vi "count rate.vi"() -> ()   [LabVIEW 2014]
doc: "This program takes in data from a Geiger counter, in order to create both a plot of the counts/interval at various times as well as a histogram. The user can select the total time and the interval over which counts should be recorded. The user can also select to omit some points since these are often junk. After counting for the selected time interval the program writes the counts vs time to a file. To create the histogram and best fit the program outputs the counts in an array to two sub vi's.\n\nBryan Ghahremani - SID: 1135515\nKenneth Heide - SID: 1269429"
uses:
  <vilib>/Platform/TimedLoop/XDataNode/timing_clust.ctl
  <vilib>/Platform/TimedLoop/XDataNode/nitl_modes.ctl
  <vilib>/Platform/TimedLoop/XDataNode/wakeup.ctl
  <vilib>/Utility/file.llb/Write To Spreadsheet File (DBL).vi
  <vilib>/platform/TimedLoop/XDataNode/XDataNode.xnode
  <vilib>/Platform/TimedLoop/XDataNode/XDNodeRunTimeDep.lvlib
panel:
  out "Decay Time":dbl=111.38825184198605
  in  "Path to Save":path
  in  "Interval (s)":dbl=1.0
  in  "?":dbl=10.0
  out "Counts vs Time":dynamicdata(graph)=[{"t0"=timestamp(0 s since 1904-01-01), "dt"=1.0, "Y"=[86.0, 89.0, 74.0, 84.0, 95.0, 101.0, 93.0, 90.0, 86.0, 91.0, 94.0, 92.0, 109.0, 103.0, 82.0, 104.0, 102.0, 122.0, 109.0, 94.0, 88.0, 105.0, 89.0, 88.0, 89.0, 85.0, 80.0, 85.0, 86.0, 89.0, 78.0, 102.0, 78.0, 80.0, 85.0, 104.0, 99.0, 81.0, 100.0, 75.0, 74.0, 80.0, 77.0, 77.0, 90.0, 73.0, 92.0, 75.0, 80.0, 80.0, 66.0, 85.0, 100.0, 99.0, 72.0, 59.0, 82.0, 106.0, 72.0, 94.0, 83.0, 70.0, 71.0, 62.0, 74.0, 83.0, 70.0, 77.0, 68.0, 78.0, 66.0, 79.0, 73.0, 79.0, 70.0, 70.0, 68.0, 58.0, 74.0, 64.0, 65.0, 67.0, 66.0, 71.0, 78.0, 55.0, 63.0, 73.0, 62.0, 58.0, 57.0, 60.0, 45.0, 63.0, 61.0, 62.0, 64.0, 56.0, 53.0, 63.0, 67.0, 63.0, 60.0, 63.0, 60.0, 51.0, 52.0, 68.0, 59.0, 50.0, 57.0, 55.0, 54.0, 45.0, 60.0, 55.0, 44.0, 66.0, 55.0, 60.0, 57.0, 53.0, 47.0, 51.0, 56.0, 49.0, 51.0, 61.0, 46.0, 61.0, 50.0, 57.0, 61.0, 47.0, 54.0, 44.0, 52.0, 57.0, 63.0, 56.0, 54.0, 56.0, 44.0, 52.0, 50.0, 48.0, 54.0, 54.0, 40.0, 47.0, 39.0, 38.0, 45.0, 48.0, 52.0, 56.0, 44.0, 47.0, 40.0, 39.0, 49.0, 43.0, 48.0, 52.0, 42.0, 48.0, 57.0, 51.0, 53.0, 34.0, 54.0, 41.0, 39.0, 42.0, 36.0, 53.0, 57.0, 43.0, 54.0, 51.0, 50.0, 56.0, 42.0, 52.0, 45.0, 34.0, 42.0, 52.0, 37.0, 59.0, 53.0, 39.0, 48.0, 46.0, 41.0, 47.0, 45.0, 42.0, 54.0, 44.0, 37.0, 38.0, 52.0, 54.0, 47.0, 44.0, 34.0, 43.0, 43.0, 45.0, 45.0, 40.0, 52.0, 48.0, 39.0, 52.0, 46.0, 49.0, 37.0, 52.0, 44.0, 42.0, 38.0, 43.0, 41.0, 40.0, 57.0, 46.0, 49.0, 39.0, 43.0, 44.0, 36.0, 41.0, 34.0, 36.0, 42.0, 45.0, 37.0, 38.0, 40.0, 52.0, 52.0, 44.0, 44.0, 47.0, 41.0, 44.0, 37.0, 35.0, 56.0, 33.0, 30.0, 41.0, 44.0, 45.0, 39.0, 47.0, 47.0, 44.0, 39.0, 41.0, 35.0, 35.0, 49.0, 59.0, 35.0, 35.0, 51.0, 36.0, 36.0, 36.0, 45.0, 36.0, 39.0, 37.0, 27.0, 35.0, 44.0, 40.0, 44.0, 41.0, 55.0, 38.0, 43.0, 37.0, 43.0, 31.0, 36.0, 28.0, 36.0]}, {"t0"=timestamp(0 s since 1904-01-01), "dt"=1.0, "Y"=array[291 elements], "attributes"=variant("NI_ChannelName"=variant(string "Best fit"))}]
  out "Histogram":dynamicdata(graph)=[{"t0"=timestamp(1 s since 1904-01-01), "dt"=2.0, "Y"=[8.352812174756966e-17, 2.888576339244969e-14, 3.1264302386873654e-12, 1.621526279731439e-10, 4.916216242584155e-09, 9.765499519537962e-08, 1.3685183070826735e-06, 1.4251050451169605e-05, 0.00011459899106855562, 0.0007330223641615576, 0.003818327119683722, 0.016510466629310206, 0.06021002372393977, 0.18767699037711996, 0.505765419365066, 1.1900692662585146, 2.4661763847755136, 4.5352483246952175, 7.451222273498955, 11.003116698148636, 14.682944866992178, 17.79266203324392, 19.666401250935436, 19.907721013027125, 18.524195754366946, 15.898522997565765, 12.625173356480483, 9.303420099997624, 6.378862242077928, 4.079700267706533, 2.4395718972978337, 1.3669389229457132, 0.7191585788466767, 0.3559392398594594, 0.16603084186175723, 0.07311461006202052, 0.030445380630477442, 0.012006094741323943, 0.004490259874679223, 0.0015948669016157635, 0.000538672357019741, 0.00017322419030295564, 5.309903520463841e-05, 1.5532655134751475e-05, 4.340604682793738e-06, 1.1599625212246946e-06, 2.9672298558293295e-07, 7.272405727293939e-08, 1.7092824738259553e-08, 3.855951772431547e-09], "attributes"=variant("NI_ChannelName"=variant(string " (Best fit)"), "NI_ExpIsRelativeTime"=variant(bool TRUE), "NI_ExpStartTimeStamp"=variant(timestamp timestamp(3500690969.465605 s since 1904-01-01)), "NI_ExpTimeStamp"=variant(timestamp timestamp(3500690969.465605 s since 1904-01-01)), "NI_ExpXDimension"=variant(string "BIN"), "NI_OriginalChannelName"=variant(string ""))}, {"t0"=timestamp(1 s since 1904-01-01), "dt"=2.0, "Y"=[0.0, 0.0, 0.0, 0.0, 0.0, 0.0, 0.0, 0.0, 0.0, 0.0, 0.0, 0.0, 0.0, 1.0, 2.0, 1.0, 5.0, 6.0, 21.0, 9.0, 21.0, 8.0, 29.0, 9.0, 15.0, 6.0, 27.0, 5.0, 17.0, 4.0, 12.0, 6.0, 7.0, 2.0, 7.0, 2.0, 9.0, 2.0, 7.0, 2.0, 8.0, 2.0, 8.0, 0.0, 8.0, 1.0, 6.0, 1.0, 0.0, 2.0], "attributes"=variant("NI_ChannelName"=variant(string " (Histogram)"), "NI_ExpIsRelativeTime"=variant(bool TRUE), "NI_ExpStartTimeStamp"=variant(timestamp timestamp(3500690969.465605 s since 1904-01-01)), "NI_ExpTimeStamp"=variant(timestamp timestamp(3500690969.465605 s since 1904-01-01)), "NI_ExpXDimension"=variant(string "BIN"), "NI_OriginalChannelName"=variant(string ""))}]
  in  "Time(s)":dbl=300.0
  out "counts per x second(s)":dbl(knob)=36.0 scale=0.0..100.0
  in  "stop":bool
  # "Omitted initial points"
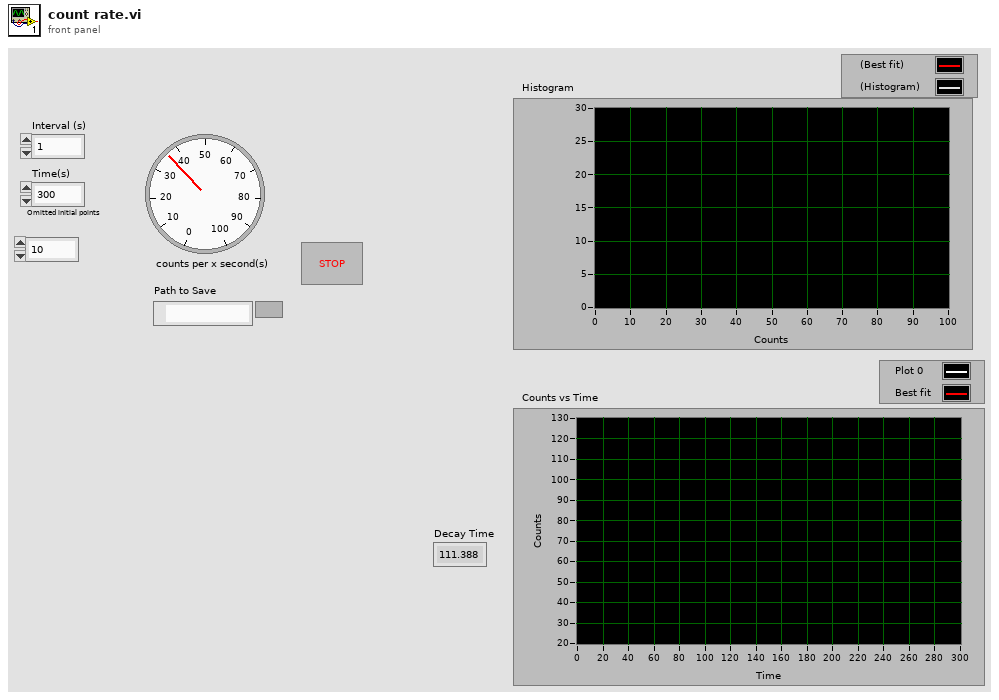
[diagram p1: front panel]
types:
  T1 = typedef "XDNodeRunTimeDep.lvlib/timing_clust.ctl" = cluster{"Expected End [f-1]":u64, "Actual End [f-1]":u64, "Finished Late? [f-1]":bool, "Expected End [i-1]":u64, "Actual End [i-1]":u64, "Finished Late? [i-1]":bool, "Expected Start [i]":u64, "Actual Start [i]":u64, "Expected Start [f]":u64, "Actual Start [f]":u64, "Source Name":string, "Structure Name":string, "Period":i64, "Deadline":i64, "Offset":i64, "Start":i64, "Priority":i32, "Timeout":i32, "Mode":T2, "Wakeup Reason":T3, "Error":errorcluster, "Source Type":string, "Secondary Source Type":string, "Global End Time":u64, "Global Start Time":u64, "Frame Duration":u64, "Iteration Duration":u64, "Assigned CPU":i32, "I/O Scan Engine Mode":u32}
  T2 = typedef "XDNodeRunTimeDep.lvlib/nitl_modes.ctl" = enum32{"No Change", "Process missed periods, maintain original phase", "Discard missed periods, maintain original phase", "Process missed periods, ignore original phase", "Discard missed periods, ignore original phase"}
  T3 = typedef "XDNodeRunTimeDep.lvlib/wakeup.ctl" = enum32{"Normal", "Aborted", "Asynchronous wakeup", "Timing source error", "Timed loop error", "Timeout"}
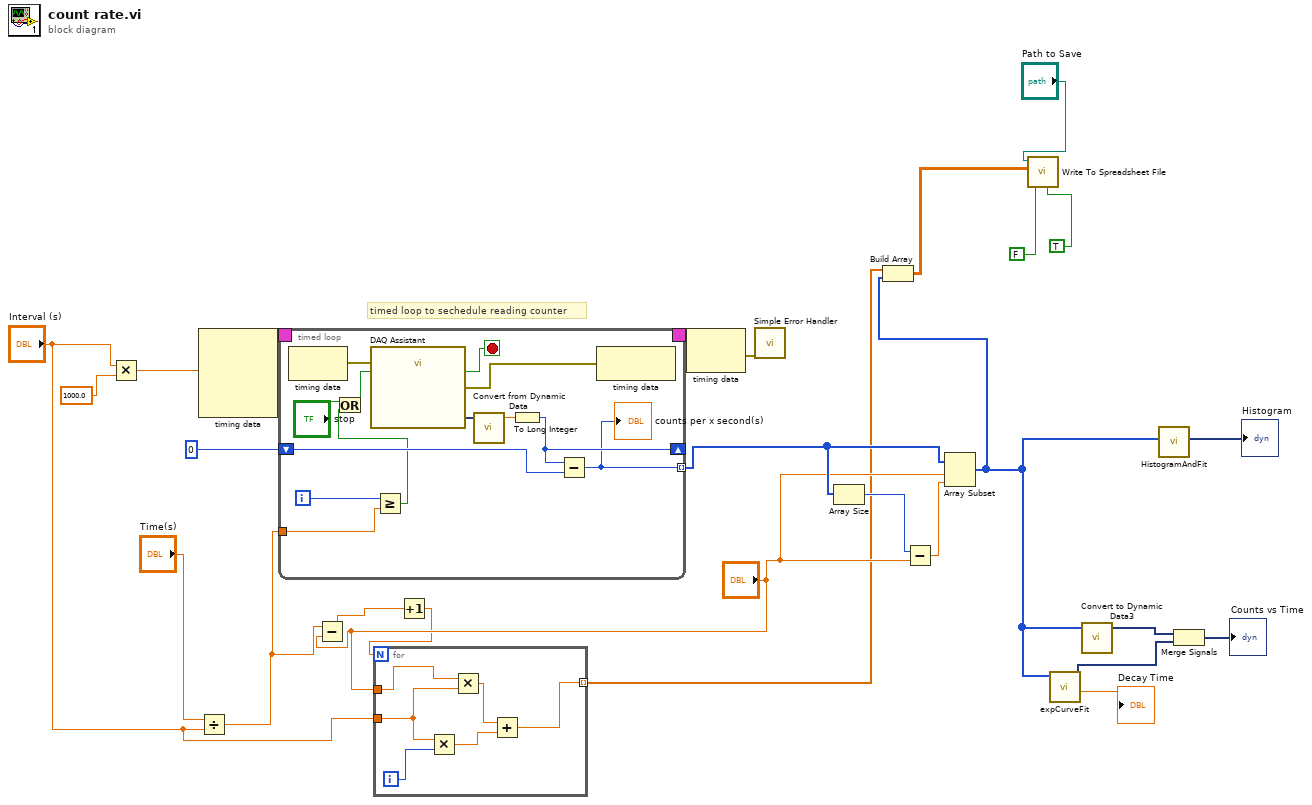
[diagram p0: block diagram]
diagram:
  # "timed loop to sechedule reading counter"
  n1 = Multiply(x="Interval (s)", y=1000.0) -> (x*y=w16:dbl)
  n2 = node-c288(w16) -> (w26:T1)  [unwired: 3 in]
  n3 = Divide(x="Time(s)", y="Interval (s)") -> (x/y=w8:dbl)
  n4 = timed-loop {
    timing: w26 -> [_]
    timing-out: [_] -> w25
    shift-right: [w36] -> _
    shift-left: 0 -> [w38]
    tunnel: w8 -> [w31]
    tunnel: [w27] -> w20 mode=indexing
    i -> [w32]
    stop <- w37 stop-if-true
    n5 = node-c288() -> (w33:errorcluster)  [unwired: 1 in]
    n6 = Greater Or Equal?(x=w32, y=w31) -> (x >= y?=w30:bool)
    n7 = Or(x="stop", y=w30) -> (x .or. y?=w28:bool)
    n8 = call "DAQ Assistant"("error in"=w33, "stop (F)"=w28) -> ("data"=w39:dynamicdata, "stopped"=w37:bool, "error out"=w34:errorcluster)  [unwired: 14 in, 1 out]
    n9 = call "Convert from Dynamic Data"("Dynamic Data Type"=w39) -> ("Scalar"=w35:dbl)  [unwired: 3 in]
    n10 = To Long Integer(number=w35) -> (32bit integer=w36:i32)
    n11 = Subtract(x=w36, y=w38) -> (x-y=w27:i32)
    "counts per x second(s)" <- w27
    n12 = node-c288(w34) -> ()  [unwired: 1 out]
  }
  n13 = Subtract(x=w8, y="?") -> (x-y=w3:dbl)
  n14 = Increment(x=w3) -> (x+1=w2:dbl)
  n15 = for {
    N: w2 -> [_]
    tunnel: "Interval (s)" -> [w47]
    tunnel: "?" -> [w48]
    tunnel: [w45] -> w5 mode=indexing
    i -> [w50]
    n16 = Multiply(x=w47, y=w50) -> (x*y=w49:dbl)
    n17 = Multiply(x=w48, y=w47) -> (x*y=w46:dbl)
    n18 = Add(x=w46, y=w49) -> (x+y=w45:dbl)
  }
  n19 = node-c288(w25) -> (w24:errorcluster)
  n20 = call <vilib>:"Simple Error Handler.vi"("error in (no error)"=w24) -> ()  [unwired: 4 in, 5 out]
  n21 = Array Size(array=w20) -> (size(s)=w19:i32)
  n22 = Subtract(x=w19, y="?") -> (x-y=w18:dbl)
  n23 = Array Subset(array=w20, index="?", length=w18) -> (w6:i32[])
  n24 = Build Array(w5, w6) -> (w4:dbl[][])
  n25 = call-poly <vilib>:"Write To Spreadsheet File.vi"("transpose? (no:F)"=TRUE, "append to file? (new file:F)"=FALSE, "2D data"=w4, "file path (dialog if empty)"="Path to Save") -> ()  [unwired: 4 in, 1 out]
  n26 = call "expCurveFit.vi"("Array"=w6) -> ("Decay Time"=→"Decay Time":dbl, "best fit"=w12:dynamicdata)  [unwired: 9 in]
  n27 = call "Convert to Dynamic Data3"("Array"=w6) -> ("Dynamic Data Type"=w21:dynamicdata)  [unwired: 3 in]
  n28 = call "HistogramAndFit.vi"("Array"=w6) -> ("Waveform Graph"=→"Histogram":dynamicdata)  [unwired: 10 in]
  n29 = Merge Signals(w21, w12) -> (→"Counts vs Time":dynamicdata)
